vi "WFS Set Aoi.vi"(6 "AOI Size Y mm":dbl, 7 "AOI Size X mm":dbl, 8 "error in (no error)":errorcluster {"code" format="%.0x"}, 9 "AOI Center Y mm":dbl, 10 "AOI Center X mm":dbl, 11 "instrument handle":refnum<visa-resource-name>) -> (0 "error out":errorcluster {"code" format="%.0x"}, 3 "instrument handle out":refnum<visa-resource-name>)   [LabVIEW 2020]
doc: "This VI defines the area of interest (AOI) within the camera image in position and size. All spots outside this area are ignored for Zernike and wavefront calculations.\n\nIn order to set the max. available area set all 4 input values to 0.0."
uses:
  WFS_32.dll
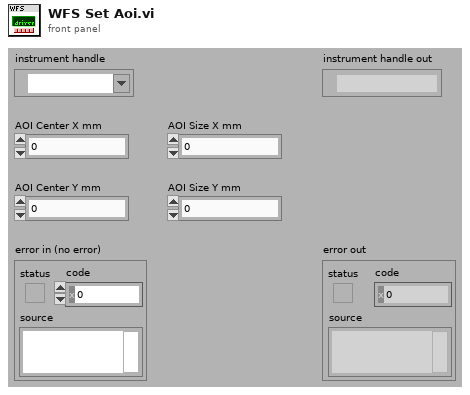
[diagram p1: front panel]
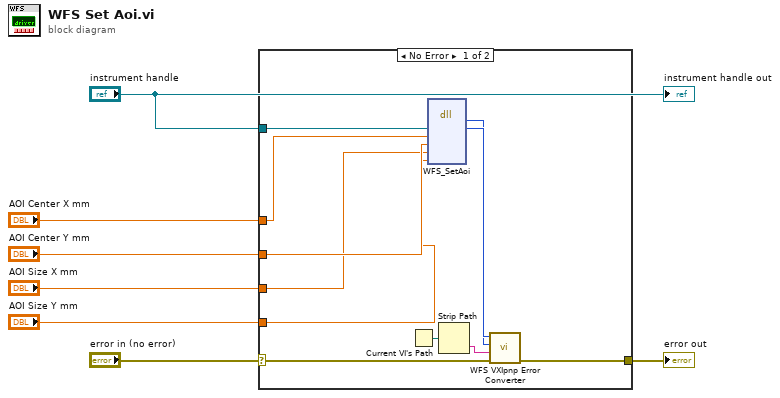
[diagram p0: block diagram]
diagram:
  n1 = case shown="No Error" "error in (no error)" {
    selector: "error in (no error)" -> [w13 w19]
    tunnel: [w12 w19] -> w7
    tunnel: "instrument handle" -> [w17 _]
    tunnel: "AOI Center X mm" -> [w11 _]
    tunnel: "AOI Center Y mm" -> [w10 _]
    tunnel: "AOI Size X mm" -> [w9 _]
    tunnel: "AOI Size Y mm" -> [w8 _]
    frame No Error {
      n2 = Current VI's Path() -> (path=w18:path)
      n3 = dll-call lib="WFS_*.*" fn="WFS_SetAoi"("Instrument Handle"=w17, "AOI Center X mm"=w11, "AOI Center Y mm"=w10, "AOI Size X mm"=w9, "AOI Size Y mm"=w8) -> (w15:i32, "Instrument Handle"=w16:u32)  [unwired: 7 in, 2 out]
      n4 = Strip Path(path=w18) -> (name=w14:string)  [unwired: 1 out]
      n5 = call "WFS VXIpnp Error Converter.vi"("error in (no error)"=w13, "Name Of VI (\"\")"=w14, "CVI Error Code (0)"=w15, "instrument handle"=w16) -> ("error out"=w12:errorcluster)  [unwired: 6 in, 1 out]
    }
    frame Error {
    }
  }
  "error out" <- w7
  "instrument handle out" <- "instrument handle"
